vi "test_Placeholder (One) Argument (Zero).vi"(8 "error in (no error)":errorcluster, 11 "TestCase in":refnum<class "Test-Layout (JSON).lvclass">=refnum) -> (0 "error out":errorcluster, 3 "TestCase out":refnum<class "Test-Layout (JSON).lvclass">)   [LabVIEW 2019, in "Test-Layout (JSON).lvclass"]
uses:
  Test-Layout (JSON).lvclass
  Layouts/JSONLayout/JSONLayout.lvclass
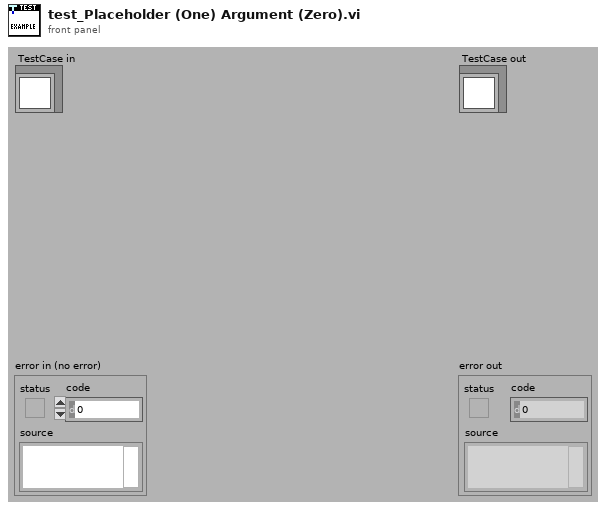
[diagram p1: front panel]
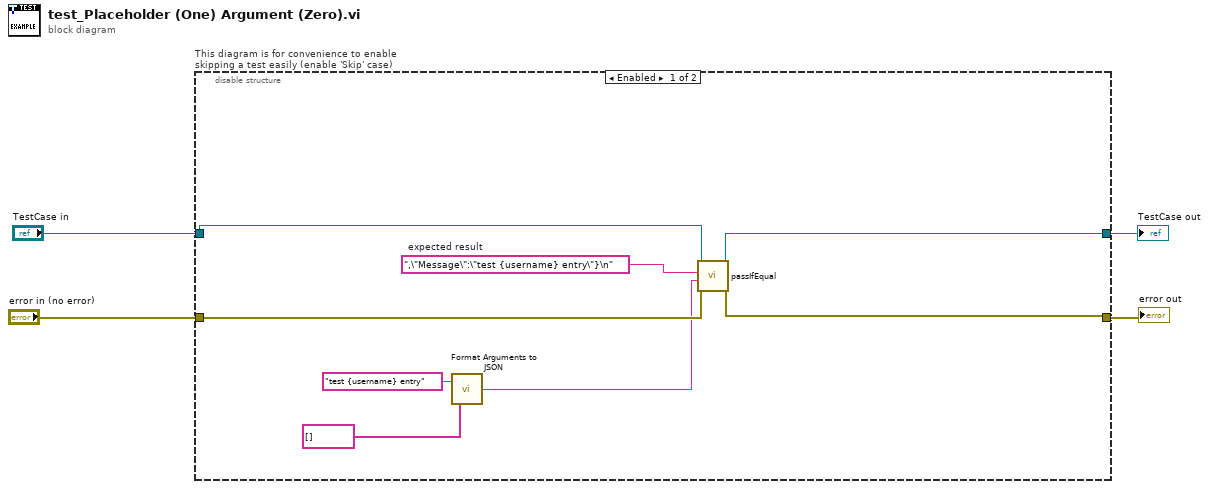
[diagram p0: block diagram]
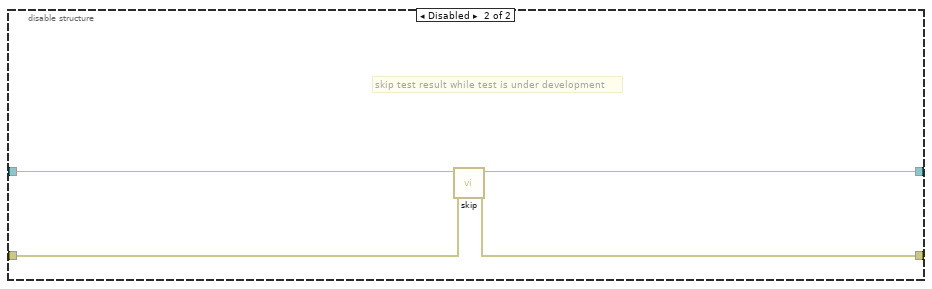
[diagram p2: hidden frame]
diagram:
  n1 = disable-structure "This diagram is for convenience to enable skipping a test easily (enable 'Skip' case)" shown="Enabled" {
    disable-tunnel: "TestCase in" -> [w11 w16]
    disable-tunnel: [w10 w14] -> w1
    disable-tunnel: [w9 w15] -> w3
    disable-tunnel: "error in (no error)" -> [w8 w13]
    frame Enabled {
      w12 = ",\"Message\":\"test {username} entry\"}\n"  # expected result
      n2 = call "Format Arguments to JSON.vi"("Arguments"=string[] [], "Message"="test {username} entry") -> ("Output Message"=w5:string)
      n3 = call-dynamic "passIfEqual.vi"("error in (no error)"=w8, "y"=w5, "x"=w12, "TestCase in"=w11) -> ("error out"=w9:errorcluster, "TestCase out"=w10:refnum<class "Test-Layout (JSON).lvclass">)  [unwired: 6 in]
    }
    frame Disabled {
      # "skip test result while test is under development"
      n4 = call <vilib>:"skip.vi"("error in (no error)"=w13, "TestCase in"=w16) -> ("error out"=w15:errorcluster, "TestCase out"=w14:refnum<class "Test-Layout (JSON).lvclass">)  [unwired: 8 in]
    }
  }
  "error out" <- w3
  "TestCase out" <- w1
